vi "rqcAlice ServiceNET Send Data.vi"(8 "error in":errorcluster, 10 "Data":u32[](array[numeric]), 11 "rqcAlice ServiceNET in":T1) -> (0 "error out":errorcluster, 3 "rqcAlice ServiceNET out":T1)   [LabVIEW 2019]
uses:
  Custom Controls/rqcAlice ServiceNET control.ctl
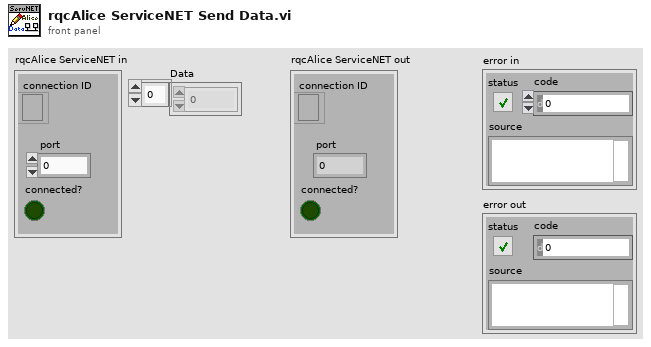
[diagram p1: front panel]
types:
  T1 = typedef "rqcAlice ServiceNET control.ctl" = cluster{"connection ID":refnum<k5>, "port":u16, "connected?":bool}
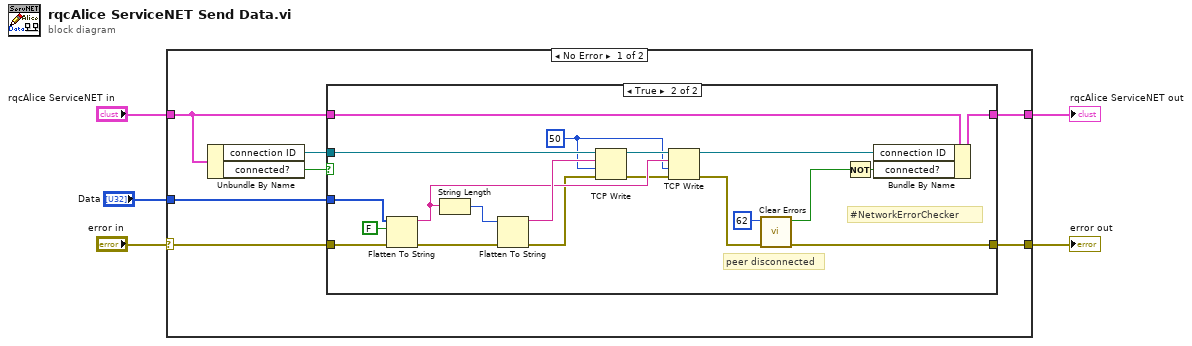
[diagram p0: block diagram]
diagram:
  n1 = case shown="No Error" "error in" {
    selector: "error in" -> [w10 w36]
    tunnel: [w9 w36] -> w4
    tunnel: "rqcAlice ServiceNET in" -> [w6 w35]
    tunnel: [w8 w35] -> w2
    tunnel: "Data" -> [w7 _]
    frame No Error {
      n2 = Unbundle By Name(w6) -> ("connection ID"=w11:refnum<k5>, "connected?"=w12:bool)
      n3 = case shown="True" w12 {
        tunnel: w11 -> [_ w34]
        tunnel: w10 -> [w14 w33]
        tunnel: [w14 w18] -> w9
        tunnel: [w13 w22] -> w8
        tunnel: w6 -> [w13 w23]
        tunnel: w7 -> [_ w19]
        frame False {
        }
        frame True {
          w20 = 50 ("timeout ms (25000)")
          # "peer disconnected"
          # "#NetworkErrorChecker"
          n4 = Flatten To String(anything=w19, prepend array or string size? (T)=FALSE, error in (no error)=w33) -> (data string=w28:string, error out=w31:errorcluster)  [unwired: 1 in, 1 out]
          n5 = String Length(string=w28) -> (length=w30:i32)
          n6 = Flatten To String(anything=w30, error in (no error)=w31) -> (data string=w29:string, error out=w27:errorcluster)  [unwired: 2 in, 1 out]
          n7 = TCP Write(connection ID=w34, data in=w29, error in (no error)=w27, 9:w20) -> (connection ID out=w25:refnum<k5>, error out=w26:errorcluster)  [unwired: 1 out]
          n8 = TCP Write(connection ID=w25, data in=w28, error in (no error)=w26, 9:w20) -> (connection ID out=w21:refnum<k5>, error out=w24:errorcluster)  [unwired: 1 out]
          n9 = call <vilib>:"Clear Errors.vi"("error in (no error)"=w24, "specific error code to clear (0: all)"=62) -> ("error out"=w18:errorcluster, "specific error cleared?"=w16:bool)  [unwired: 4 in]
          n10 = Not(x=w16) -> (.not. x?=w15:bool)
          n11 = Bundle By Name(cluster=w23, "connection ID"=w21, "connected?"=w15) -> (w22:T1)
        }
      }
    }
    frame Error {
    }
  }
  "rqcAlice ServiceNET out" <- w2
  "error out" <- w4
